vi "Subscribe & Monitor ERD.vi"(7 "Subscription Timeout (s)":i32=10, 8 "Error In":errorcluster, 9 "ERD to Subscribe To":T2 {"ERD Number" format="%.0x"}, 10 "GEA Inputs":T1={"Source"=228, "Destination"=0} {"Destination" format="%.0x"; "Source" format="%.0x"}, 11 "GEA2 Reference In":refnum<k24>) -> (0 "Error Out":errorcluster, 1 "Current ERD Data":string, 2 "Array - String":string[](array[string]), 3 "GEA2 Reference Out":refnum<k24>)   [LabVIEW 2016, in "TLMB.lvlib"]
uses:
  Projects/TLMB.lvlib
  Common/LabVIEW GEA2 Toolkit/LabVIEW_GEA2_Toolkit.lvlibp/type defs/ERD Read Data In.ctl
  Common/LabVIEW GEA2 Toolkit/LabVIEW_GEA2_Toolkit.lvlibp/type defs/Data Type.ctl
  Common/LabVIEW GEA2 Toolkit/LabVIEW_GEA2_Toolkit.lvlibp/type defs/Source_Destination.ctl
  Q:/Common/DLLs/GEA3/GeaCommunication.dll
  Common/DLLs/GEA3/GeaCommunication.dll
  Common/LabVIEW GEA2 Toolkit/LabVIEW_GEA2_Toolkit.lvlibp/type defs/Data In.ctl
  Common/LabVIEW GEA2 Toolkit/LabVIEW_GEA2_Toolkit.lvlibp
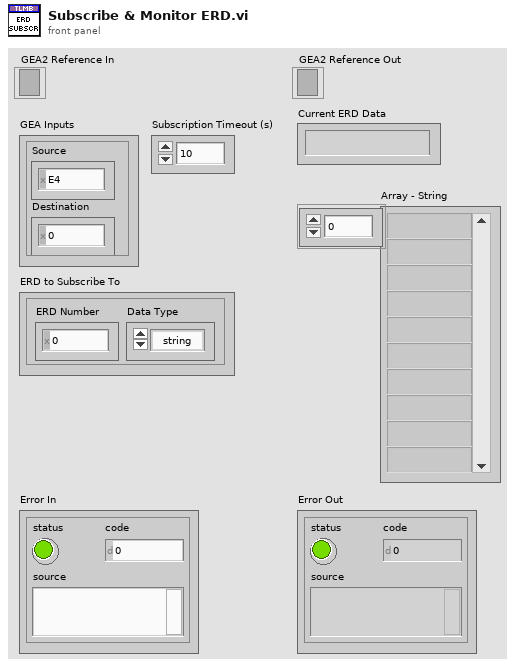
[diagram p1: front panel]
types:
  T1 = typedef "LabVIEW_GEA2_Toolkit.lvlibp/Source_Destination.ctl" = cluster{"Source":u8, "Destination":u8}
  T2 = typedef "LabVIEW_GEA2_Toolkit.lvlibp/ERD Read Data In.ctl" = cluster{"ERD Number":u16, "Data Type":T3}
  T3 = typedef "LabVIEW_GEA2_Toolkit.lvlibp/Data Type.ctl" = enum16{"string", "boolean", "uint8_t", "uint16_t", "uint32_t", "uint64_t", "int8_t", "int16_t", "int32_t", "int64_t"}
  T4 = typedef "LabVIEW_GEA2_Toolkit.lvlibp/Data In.ctl" = cluster{"Source":u8, "Destination":u8, "Command":u8, "Message":string}
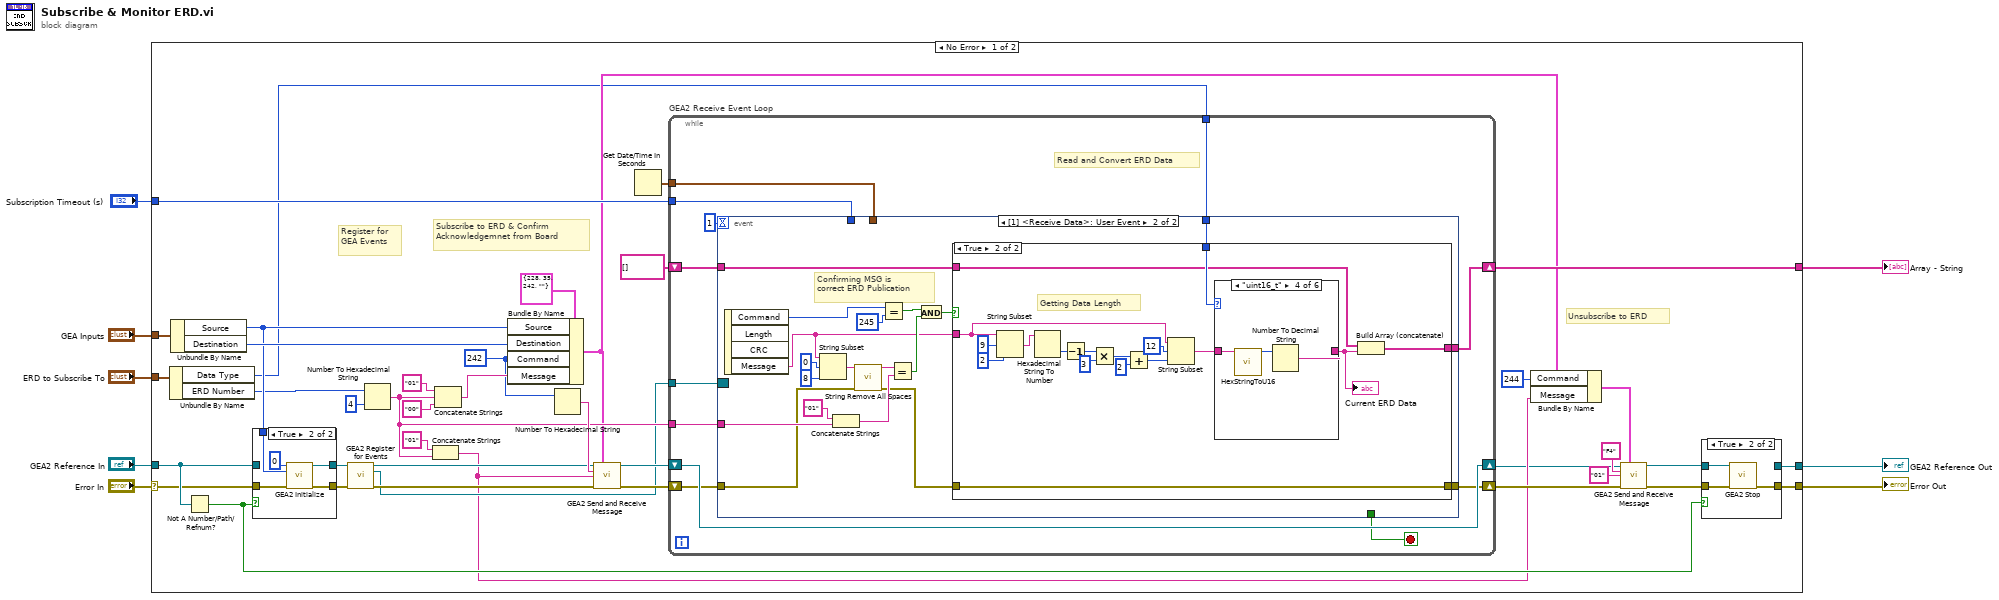
[diagram p0: block diagram]
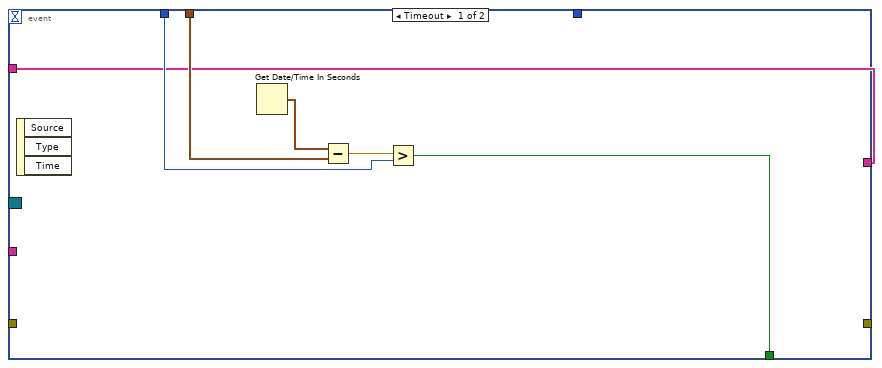
[diagram p2: hidden frame]
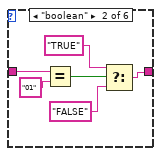
[diagram p5: hidden frame]
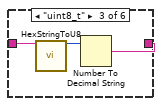
[diagram p6: hidden frame]
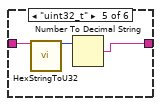
[diagram p7: hidden frame]
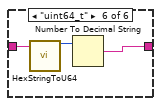
[diagram p8: hidden frame]
diagram:
  n1 = case shown="No Error" "Error In" {
    selector: "Error In" -> [w21 w138]
    tunnel: "GEA Inputs" -> [w48 _]
    tunnel: "ERD to Subscribe To" -> [w46 _]
    tunnel: "GEA2 Reference In" -> [w39 w137]
    tunnel: [w37 w138] -> w5
    tunnel: "Subscription Timeout (s)" -> [w27 _]
    tunnel: [w25 w137] -> w3
    tunnel: [w22 _] -> w1
    frame No Error {
      w42 = u8 242 ("Command")
      # "Unsubscribe to ERD"
      # "Register for\nGEA Events"
      # "Subscribe to ERD & Confirm \nAcknowledgemnet from Board"
      n2 = Unbundle By Name(w46) -> ("Data Type"=w14:T3, "ERD Number"=w13:u16)
      n3 = Unbundle By Name(w48) -> ("Source"=w38:u8, "Destination"=w47:u8)
      n4 = Not A Number/Path/Refnum?(number/path/refnum=w39) -> (NaN/Path/Refnum?=w36:bool)
      n5 = case shown="True" w36 {
        tunnel: [w131 w135] -> w33
        tunnel: w39 -> [w131 _]
        tunnel: [w130 w136] -> w35
        tunnel: w38 -> [_ w133]
        tunnel: w21 -> [w130 w132]
        frame False {
        }
        frame True {
          n6 = call "GEA2 Initialize.vi"("Board Index"=0, "Source Address"=w133, "error in"=w132) -> ("GEA2 Reference Out"=w135:refnum<k24>, "error out"=w136:errorcluster)  [unwired: 10 in, 1 out]
        }
      }
      n7 = call "GEA2 Register for Events.vi"("GEA2 Reference In"=w33, "Error In"=w35) -> ("GEA2 Reference Out"=w32:refnum<k24>, "Event Registration Refnum"=w26:refnum<event-registration>, "Error Out"=w34:errorcluster)  [unwired: 11 in]
      n8 = Number To Hexadecimal String(1:i16 4 ("width (-)"), 2:w13) -> (0:w28:string)
      n9 = Concatenate Strings("01" ("string"), w28) -> (w15:string)
      n10 = Concatenate Strings("01" ("string"), w28, "00" ("string")) -> (w43:string)
      n11 = Bundle By Name(cluster=T4 {"Source"=228, "Destination"=35, "Command"=242, "Message"=""} ("Input Data"), "Source"=w38, "Destination"=w47, "Command"=w42, "Message"=w43) -> (w17:T4)
      n12 = Number To Hexadecimal String(2:w42) -> (0:w41:string)  [unwired: 1 in]
      n13 = call "GEA2 Send and Receive Message.vi"("GEA2 Reference In"=w32, "Input Data"=w17, "Expected Command"=w41, "Expected Data"=w15, "Error In"=w34) -> ("GEA2 Reference Out"=w30:refnum<k24>, "Error Out"=w31:errorcluster)  [unwired: 7 in, 2 out]
      n14 = Get Date/Time In Seconds() -> (seconds since 1Jan1904=w24:timestamp)
      n15 = while "GEA2 Receive Event Loop" {
        tunnel: w26 -> [w58]
        shift-right: [w59] -> w29
        shift-left: w31 -> [w60]
        tunnel: w28 -> [w57]
        tunnel: w27 -> [w51]
        tunnel: w14 -> [w56]
        tunnel: w24 -> [w52]
        shift-right: [w54] -> w22
        shift-left: string[] [] -> [w55]
        shift-right: [w61] -> w11
        shift-left: w30 -> [w61]
        stop <- w50 stop-if-true
        # "Read and Convert ERD Data"
        n16 = event shown="[1] <Receive Data>: User Event" {
          selector: w58 -> [_ _]
          dyn-events: _ -> [_ _]
          timeout: 1 -> [_ _]
          tunnel: w60 -> [_ w72]
          tunnel: [_ w73] -> w59
          tunnel: w57 -> [_ w79]
          tunnel: w56 -> [_ w74]
          tunnel: w55 -> [w62 w70]
          tunnel: [w62 w69] -> w54
          tunnel: w52 -> [w66 _]
          tunnel: w51 -> [w64 _]
          tunnel: [w63 _] -> w50
          event Timeout {
            n17 = event-data() -> ()  [unwired: 1 in, 3 out]
            n18 = Get Date/Time In Seconds() -> (seconds since 1Jan1904=w67:timestamp)
            n19 = Subtract(x=w67, y=w66) -> (x-y=w65:dbl)
            n20 = Greater?(x=w65, y=w64) -> (0:w63:bool)
          }
          event User Event {
            # "Confirming MSG is\ncorrect ERD Publication"
            n21 = event-data() -> ("Command"=w81:u8, "Message"=w68:string)  [unwired: 1 in, 2 out]
            n22 = String Subset(string=w68, offset (0)=0, length (rest)=8 ("length (rest)")) -> (substring=w76:string)
            n23 = Concatenate Strings("01" ("string"), w79) -> (w84:string)
            n24 = call "String Remove All Spaces.vi"("Input String"=w76, "error in (no error)"=w72) -> ("Spaces Removed"=w75:string, "error out"=w71:errorcluster)  [unwired: 12 in]
            n25 = Equal?(x=w81, y=u8 245) -> (x = y?=w85:bool)
            n26 = Equal?(x=w75, y=w84) -> (x = y?=w86:bool)
            n27 = And(x=w85, y=w86) -> (x .and. y?=w80:bool)
            n28 = case shown="True" w80 {
              tunnel: w68 -> [_ w95]
              tunnel: w74 -> [_ w94]
              tunnel: w71 -> [w88 w92]
              tunnel: [w88 w92] -> w73
              tunnel: w70 -> [w87 w91]
              tunnel: [w87 w89] -> w69
              frame False {
              }
              frame True {
                # "Getting Data Length"
                n29 = String Subset(string=w95, offset (0)=9, length (rest)=2 ("length (rest)")) -> (substring=w103:string)
                n30 = Hexadecimal String To Number(string=w103) -> (number=w101:u32)  [unwired: 2 in, 1 out]
                n31 = Decrement(x=w101) -> (x-1=w102:u32)
                n32 = Multiply(x=w102, y=u32 3) -> (x*y=w99:u32)
                n33 = Add(x=w99, y=u32 2) -> (x+y=w97:u32)
                n34 = String Subset(string=w95, offset (0)=12, length (rest)=w97) -> (substring=w93:string)
                n35 = case shown="\"uint16_t\"" w94 {
                  tunnel: w93 -> [w106 w112 w115 w118 w120 w124]
                  tunnel: [w106 w107 w113 w116 w121 w122] -> w90
                  frame "string", Default {
                  }
                  frame "boolean" {
                    n36 = Equal?(x=w112, y="01") -> (x = y?=w110:bool)
                    n37 = Select(t="TRUE", s=w110, f="FALSE") -> (s? t:f=w107:string)
                  }
                  frame "uint8_t" {
                    n38 = call "HexStringToU8.vi"("Input String"=w115) -> ("Number Out"=w114:u8)  [unwired: 14 in]
                    n39 = Number To Decimal String(number=w114) -> (decimal integer string=w113:string)  [unwired: 1 in]
                  }
                  frame "uint16_t" {
                    n40 = call "HexStringToU16.vi"("Input String"=w118) -> ("Number Out"=w117:u16)  [unwired: 14 in]
                    n41 = Number To Decimal String(number=w117) -> (decimal integer string=w116:string)  [unwired: 1 in]
                  }
                  frame "uint32_t" {
                    n42 = call "HexStringToU32.vi"("Input String"=w120) -> ("Number Out"=w119:u32)  [unwired: 14 in]
                    n43 = Number To Decimal String(number=w119) -> (decimal integer string=w121:string)  [unwired: 1 in]
                  }
                  frame "uint64_t" {
                    n44 = call "HexStringToU64.vi"("Input String"=w124) -> ("Number Out"=w123:u64)  [unwired: 14 in]
                    n45 = Number To Decimal String(number=w123) -> (decimal integer string=w122:string)  [unwired: 1 in]
                  }
                }
                "Current ERD Data" <- w90
                n46 = Build Array (concatenate)(w91, w90) -> (w89:string[])
              }
            }
          }
        }
      }
      n47 = Bundle By Name(cluster=w17, "Command"=u8 244, "Message"=w15) -> (w12:T4)
      n48 = call "GEA2 Send and Receive Message.vi"("GEA2 Reference In"=w11, "Input Data"=w12, "Expected Command"="F4", "Expected Data"="01", "Error In"=w29) -> ("GEA2 Reference Out"=w10:refnum<k24>, "Error Out"=w20:errorcluster)  [unwired: 7 in, 2 out]
      n49 = case shown="True" w36 {
        tunnel: [w126 w129] -> w37
        tunnel: w10 -> [w125 w128]
        tunnel: w20 -> [w126 w127]
        tunnel: [w125 _] -> w25
        frame False {
        }
        frame True {
          n50 = call "GEA2 Stop.vi"("GEA2 Reference In"=w128, "Error In"=w127) -> ("Error Out"=w129:errorcluster)  [unwired: 13 in]
        }
      }
    }
    frame Error {
    }
  }
  "Error Out" <- w5
  "GEA2 Reference Out" <- w3
  "Array - String" <- w1
